vi "median and average.vi"(0 "sensor 1":void[](array[numeric]), 1 "sensor2":void[](array[numeric]), 2 "sensor3":void[](array[numeric]), 3 "sensor 4":void[](array[numeric]), 4 "sensor 5":void[](array[numeric]), 5 "sensor 6":void[](array[numeric]), 6 "sensor 7":void[](array[numeric]), 7 "sensor 8":void[](array[numeric]), 9 "sensor 9":void[](array[numeric])) -> ()   [LabVIEW 2017]
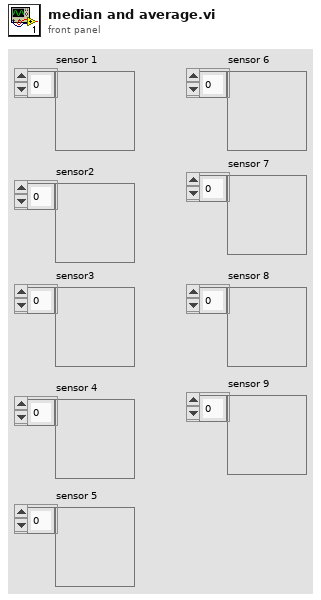
[diagram p1: front panel]
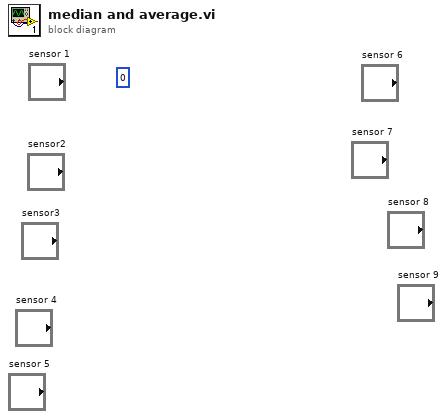
[diagram p0: block diagram]
diagram:
  (unwired) 0
